vi "synnax writer close.vi"(8 "error in":errorcluster, 11 "writer handle":u64) -> (0 "error out":errorcluster)   [LabVIEW 2026, in "synnax_clib.lvlib" / "Synnax Writer.lvclass"]
uses:
  Synnax Writer.lvclass
  synnax_clib.dll
  synnax_clib.lvlib
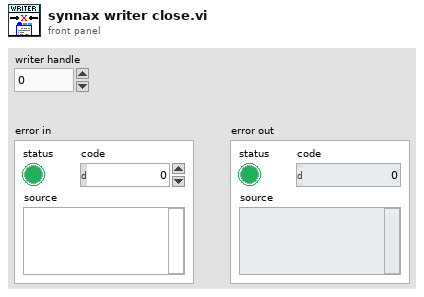
[diagram p1: front panel]
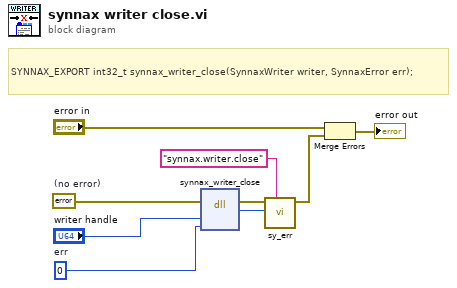
[diagram p0: block diagram]
diagram:
  w2 = errorcluster {"status"=FALSE, "code"=0, "source"=""}  # (no error)
  w9 = u64 0  # err
  # "SYNNAX_EXPORT int32_t synnax_writer_close(SynnaxWriter writer, SynnaxError err);"
  n1 = dll-call lib="C/synnax/client/labview/synnax_clib.*" fn="synnax_writer_close"(error in=w2, "writer"="writer handle", "err"=w9) -> (error out=w8:errorcluster, w7:i32)  [unwired: 4 in, 1 out]
  n2 = call "sy_err.vi"("source"="synnax.writer.close", "error code"=w7, "error in (no error)"=w8) -> ("error out"=w3:errorcluster)  [unwired: 8 in]
  n3 = Merge Errors("error in", w3) -> (→"error out":errorcluster)
